vi "Start Stream.vi"(8 "error in (no error)":errorcluster, 11 "Red Pitaya Digitizer in":refnum<class "Red Pitaya Digitizer.lvclass">) -> (0 "error out":errorcluster, 3 "Red Pitaya Digitizer out":refnum<class "Red Pitaya Digitizer.lvclass">)   [LabVIEW 2016, in "Red Pitaya Digitizer.lvclass"]
uses:
  Red Pitaya Digitizer.lvclass
  C:/github/NHMFL_Core/Libraries/Instruments/Pulse Driver/Pulse Driver.lvclass
  C:/github/NHMFL_Core/Libraries/Instruments/Instrument Driver/Instrument Driver.lvclass
  Red Pitaya Digitizer.lvclass/Red Pitaya Digitizer.ctl
  Instruments/Pulse Driver/Pulse Driver.lvclass/Pulse Driver.ctl
  Instruments/Instrument Driver/Instrument Driver.lvclass/Instrument Driver.ctl
  Instruments/Pulse Driver/Read tdms file.vi
  Instruments/Instrument Driver/Read Group name.vi
  Instruments/Instrument Driver/Read Channel names.vi
  Instruments/Pulse Driver/Write tdms file.vi
  Instruments/Pulse Driver/Pulse Driver.lvclass
  RP Core/RP Instrument/RP Instrument.lvclass
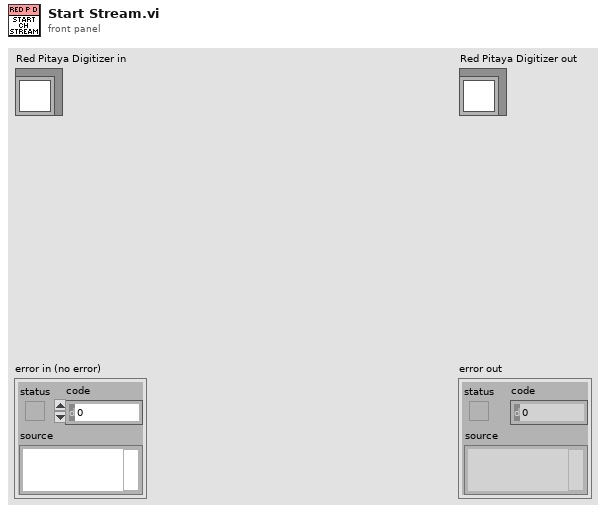
[diagram p1: front panel]
types:
  T1 = typedef "Lockin Parameters.ctl" = cluster{"Frequency":dbl, "Phase":dbl, "Syncronous":bool, "Points per sine wave":i32, "DDS":bool, "Frequency word":u32, "Phase word":u32, "DDS modulus":i64, "DDS clock":dbl}
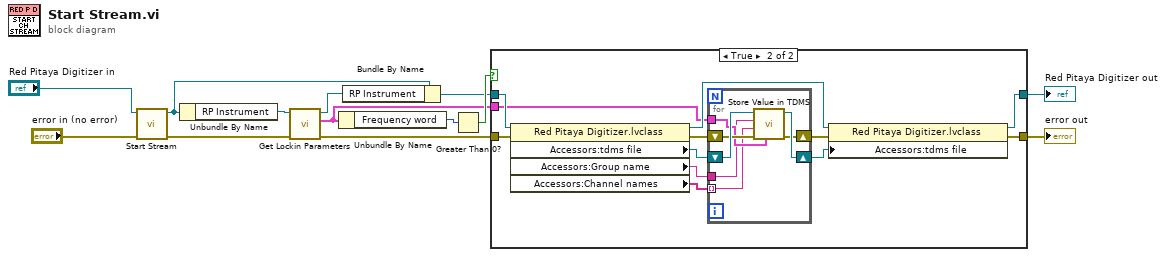
[diagram p0: block diagram]
diagram:
  n1 = call-parent "Start Stream.vi"("error in (no error)"="error in (no error)", "Pulse Driver in"="Red Pitaya Digitizer in") -> ("error out"=w9:errorcluster, "Pulse Driver out"=w8:refnum<class "Red Pitaya Digitizer.lvclass">)  [unwired: 8 in]
  n2 = Unbundle By Name(w8) -> ("RP Instrument"=w10:refnum<class "RP Instrument.lvclass">)
  n3 = call-dynamic "Get Lockin Parameters.vi"("error in (no error)"=w9, "RP Instrument in"=w10) -> ("error out"=w4:errorcluster, "Lockin parameters"=w1:T1, "RP Instrument out"=w7:refnum<class "RP Instrument.lvclass">)  [unwired: 7 in]
  n4 = Unbundle By Name(w1) -> ("Frequency word"=w11:u32)
  n5 = Bundle By Name(cluster=w8, "RP Instrument"=w7) -> (w5:refnum<class "Red Pitaya Digitizer.lvclass">)
  n6 = Greater Than 0?(x=w11) -> (x > 0?=w6:bool)
  n7 = case shown="True" w6 {
    tunnel: w5 -> [w15 w27]
    tunnel: w4 -> [w14 w25]
    tunnel: [w15 w20] -> w3
    tunnel: [w14 w19] -> w2
    tunnel: w1 -> [_ w18]
    frame False {
    }
    frame True {
      n8 = property class="Red Pitaya Digitizer.lvclass"(reference=w27, error in=w25) -> (reference out=w26:refnum<class "Red Pitaya Digitizer.lvclass">, error out=w22:errorcluster, "Accessors:tdms file"=w24:refnum<k34>, "Accessors:Group name"=w17:string, "Accessors:Channel names"=w16:string[])
      n9 = for {
        tunnel: w18 -> [w30]
        shift-right: [w33] -> w23
        shift-left: w24 -> [w34]
        shift-right: [w31] -> w21
        shift-left: w22 -> [w32]
        tunnel: w17 -> [w29]
        tunnel: w16 -> [w28] mode=indexing
        n10 = call "Store Value in TDMS.vi"("Value"=w30, "Error In"=w32, "channel name"=w28, "group name"=w29, "tdms file"=w34) -> ("Error Out"=w31:errorcluster, "tdms file out"=w33:refnum<k34>)  [unwired: 3 in, 2 out]
      }
      n11 = property class="Red Pitaya Digitizer.lvclass"(reference=w26, error in=w21, "Accessors:tdms file"=w23) -> (reference out=w20:refnum<class "Red Pitaya Digitizer.lvclass">, error out=w19:errorcluster)
    }
  }
  "error out" <- w2
  "Red Pitaya Digitizer out" <- w3
